vi "List - Reset Value.vi"(8 "Error In":errorcluster, 11 "List In":cluster{"Name":string, "Selected":bool}[](array[cluster])) -> (0 "Error Out":errorcluster, 3 "List Out":cluster{"Name":string, "Selected":bool}[](array[cluster]))   [LabVIEW 2020]
doc: "This VI use to reset the values to default values.\nDefault values is False."
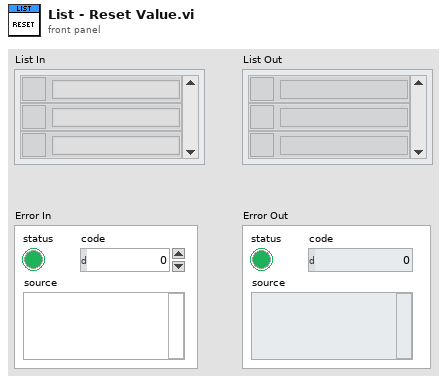
[diagram p1: front panel]
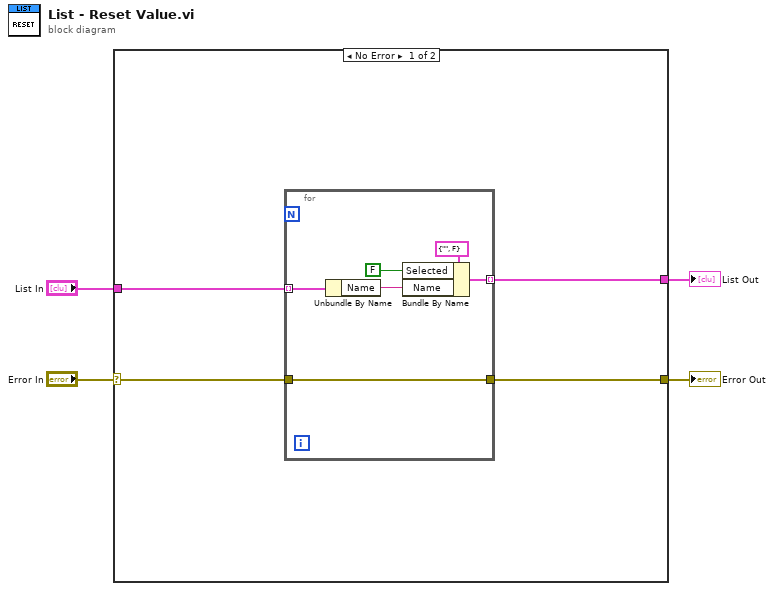
[diagram p0: block diagram]
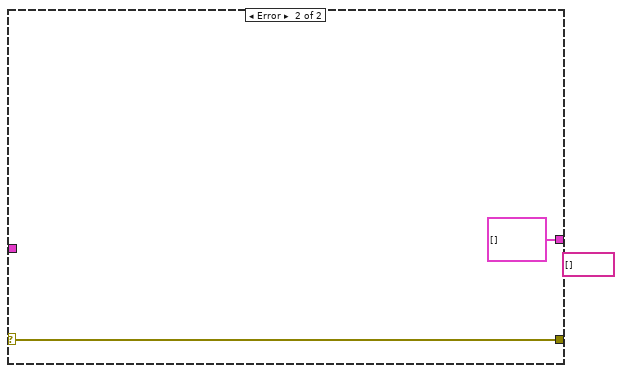
[diagram p2: hidden frame]
diagram:
  n1 = case shown="No Error" "Error In" {
    selector: "Error In" -> [w8 w16]
    tunnel: [w7 w16] -> w3
    tunnel: "List In" -> [w6 _]
    tunnel: [w5 cluster{"Name":string, "Selected":bool}[] []] -> w2
    frame No Error {
      n2 = for {
        tunnel: w6 -> [w10] mode=indexing
        tunnel: [w14] -> w7
        tunnel: w8 -> [w14]
        tunnel: [w11] -> w5 mode=indexing
        n3 = Unbundle By Name(w10) -> ("Name"=w9:string)
        n4 = Bundle By Name(cluster=cluster{"Name":string, "Selected":bool} {"Name"="", "Selected"=FALSE} ("File List"), "Selected"=FALSE, "Name"=w9) -> (w11:cluster{"Name":string, "Selected":bool})
      }
    }
    frame Error {
      (unwired) string[] []
      (unwired) string[] []
    }
  }
  "Error Out" <- w3
  "List Out" <- w2
